vi "Nuovo valore rpm.vi"() -> (1 "RPM":string, 2 "OK ?":bool)   [LabVIEW 2019]
panel:
  in  "Cancel Button":bool
  in  "OK Button":bool
  in  "NUOVO VALORE RPM":dbl
  # "MODIFICA VALORE RPM ACQUISIZIONE"
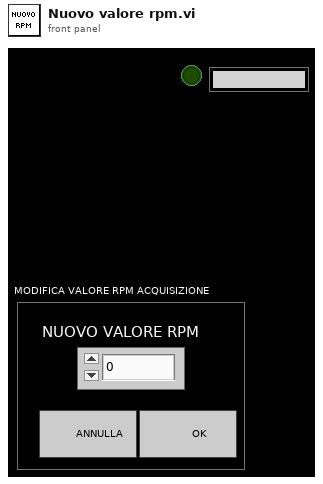
[diagram p1: front panel]
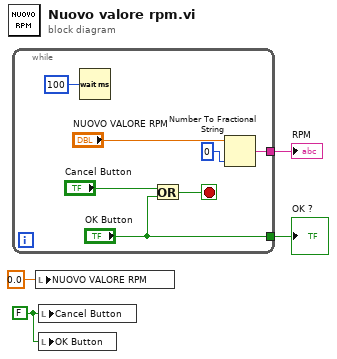
[diagram p0: block diagram]
diagram:
  w3 = FALSE ("Cancel Button")
  n1 = while {
    tunnel: ["OK Button"] -> w4
    tunnel: [w5] -> w2
    stop <- w9 stop-if-true
    n2 = Wait (ms)(milliseconds to wait=u32 100) -> ()  [unwired: 1 out]
    n3 = Or(x="Cancel Button", y="OK Button") -> (x .or. y?=w9:bool)
    n4 = Number To Fractional String(number="NUOVO VALORE RPM", precision (6)=i16 0) -> (F-format string=w5:string)  [unwired: 2 in]
  }
  "OK ?" <- w4
  "RPM" <- w2
  n5 = local write "NUOVO VALORE RPM"(0.0 ("NUOVO VALORE RPM")) -> ()
  n6 = local write "Cancel Button"(w3) -> ()
  n7 = local write "OK Button"(w3) -> ()
